vi "Entry - Generate Wash Cycle.vi"(8 "error in (no error)":errorcluster, 10 "Wash Steps":T6, 11 "View Model":T1) -> (0 "error out":errorcluster, 3 "View Model":T1)   [LabVIEW 2017]
doc: "Transform selected Wash Steps into Wash Cycle."
uses:
  Controls/Entry - Wash Steps.ctl
  View Model/Controls/View Model.ctl
  View Model/Controls/Shared Model.ctl
  Error Handler/Controls/Error Model.ctl
  Error Handler/Controls/Error Message.ctl
  Error Handler/Controls/Error Level.ctl
  Configuration/Controls/Database Model.ctl
  Configuration/Controls/Database Message.ctl
  Configuration/Controls/Database Command.ctl
  Configuration/Controls/Database Overhead.ctl
  Configuration/Controls/Database Status.ctl
  Configuration/Controls/Database Record.ctl
  Controller/Controls/CNTRLR - Model.ctl
  Controller/Controls/CNTRLR - Message.ctl
  Controller/Controls/CNTRLR - Command.ctl
  Controller/Controls/CNTRLR - Overhead.ctl
  Controller/Controls/CNTRLR - Position.ctl
  Controller/Controls/CNTRLR - State.ctl
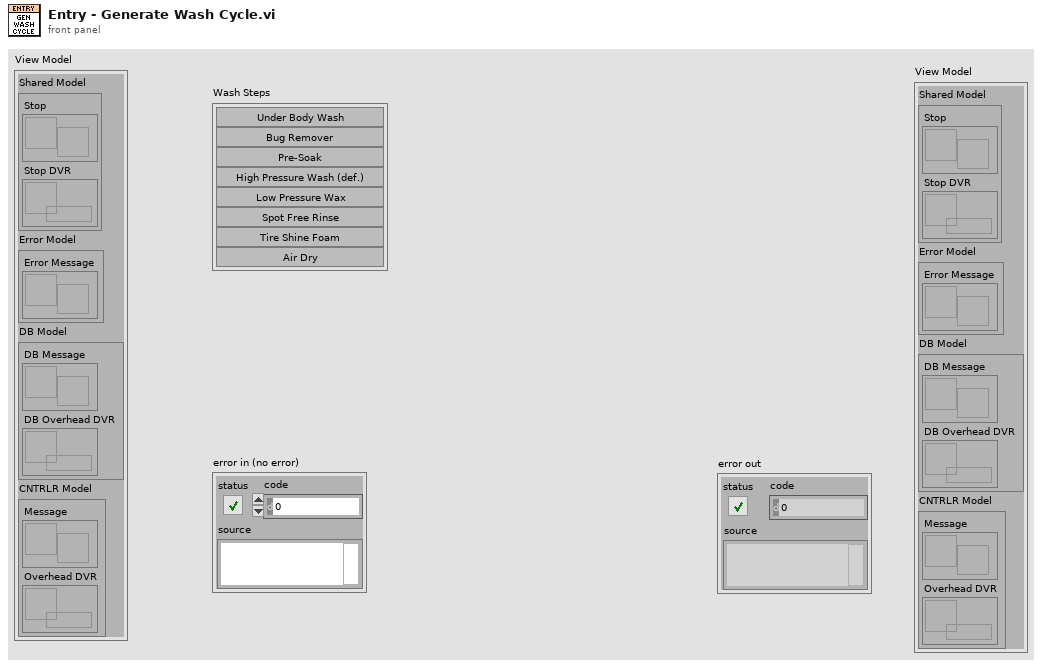
[diagram p1: front panel]
types:
  T1 = typedef "View Model.ctl" = cluster{"Shared Model":T2, "Error Model":T3, "DB Model":T4, "CNTRLR Model":T5}
  T2 = typedef "Shared Model.ctl" = cluster{"Stop":refnum<user-event>, "Stop DVR":refnum<data-value>}
  T3 = typedef "Error Model.ctl" = cluster{"Error Message":refnum<user-event>}
  T4 = typedef "Database Model.ctl" = cluster{"DB Message":refnum<user-event>, "DB Overhead DVR":refnum<data-value>}
  T5 = typedef "CNTRLR - Model.ctl" = cluster{"Message":refnum<user-event>, "Overhead DVR":refnum<data-value>}
  T6 = typedef "Entry - Wash Steps.ctl" = cluster{"Under Body Wash":bool, "Bug Remover":bool, "Pre-Soak":bool, "High Pressure Wash":bool, "Low Pressure Wax":bool, "Spot Free Rinse":bool, "Tire Shine Foam":bool, "Air Dry":bool}
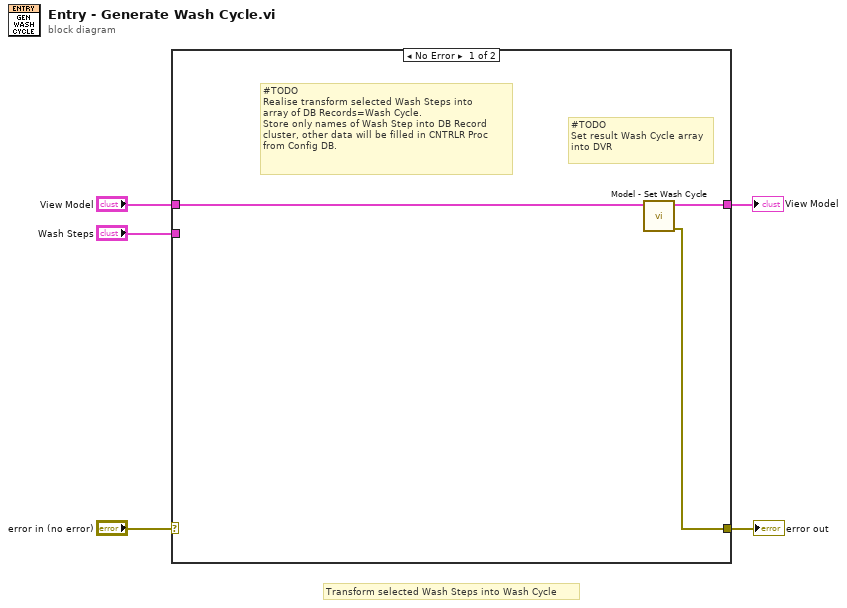
[diagram p0: block diagram]
diagram:
  # "Transform selected Wash Steps into Wash Cycle"
  n1 = case shown="No Error" "error in (no error)" {
    selector: "error in (no error)" -> [_ w10]
    tunnel: [w6 w10] -> w4
    tunnel: "Wash Steps" -> [_ _]
    tunnel: [w8 w9] -> w2
    tunnel: "View Model" -> [w7 w9]
    frame No Error {
      # "#TODO\nSet result Wash Cycle array\ninto DVR"
      # "#TODO\nRealise transform selected Wash Steps into\narray of DB Records=Wash Cycle.\nStore only names of Wash Step into DB Record\ncluster, other data will be filled in CNTRLR Proc\nfrom Config DB."
      n2 = call "Model - Set Wash Cycle.vi"("View Model"=w7) -> ("error out"=w6:errorcluster, "View Model"=w8:T1)  [unwired: 9 in]
    }
    frame Error {
    }
  }
  "error out" <- w4
  "View Model" <- w2
